vi "LsstLineDecode.vi"(11 "new lines":string) -> (0 "Chart":dbl(graph), 1 "payload":string, 2 "cmd":string, 3 "text":string, 4 "Graph":dbl[](graph))   [LabVIEW 2022 SP3]
uses:
  <vilib>/Utility/error.llb/Trim Whitespace One-Sided.vi
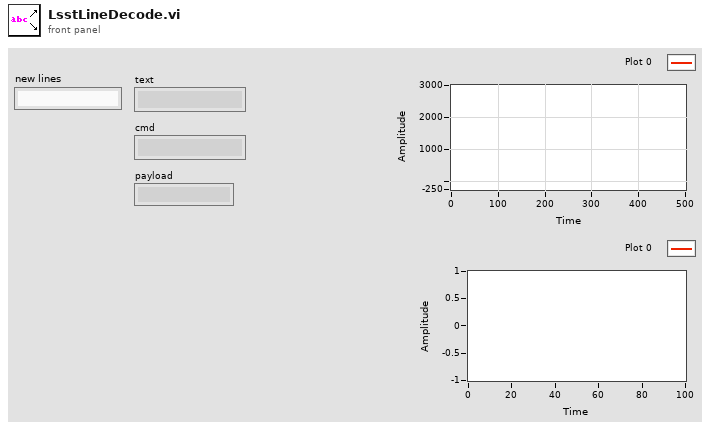
[diagram p1: front panel]
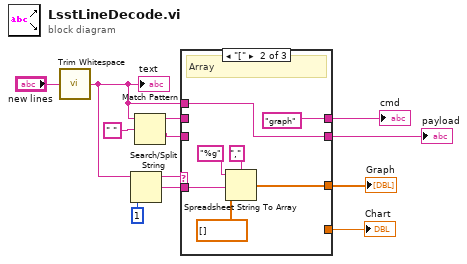
[diagram p0: block diagram]
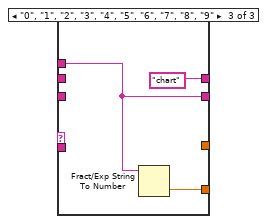
[diagram p3: hidden frame]
diagram:
  n1 = call <vilib>:"Trim Whitespace.vi"("string"="new lines") -> ("trimmed string"=w3:string)  [unwired: 1 in]
  "text" <- w3
  n2 = Search/Split String(string=w3, offset (0)=1) -> (substring before match=w5:string, match + rest of string=w4:string)  [unwired: 1 in, 1 out]
  n3 = Match Pattern(string=w3, regular expression=" ") -> (before substring=w9:string, after substring=w7:string)  [unwired: 1 in, 2 out]
  n4 = case shown="\"[\"" w5 {
    tunnel: w4 -> [_ w19 _]
    tunnel: [_ w17 _] -> w12
    tunnel: [w14 "graph" ("regular expression") "chart" ("regular expression")] -> w1
    tunnel: w9 -> [w14 _ _]
    tunnel: [w13 w15 w22] -> w8
    tunnel: w7 -> [w13 _ _]
    tunnel: w3 -> [_ w15 w22]
    tunnel: [_ _ w24] -> w2
    frame Default {
      # "not data"
    }
    frame "[" {
      # "Array"
      n5 = Spreadsheet String To Array(delimiter (Tab)=",", format string="%g", spreadsheet string=w19, array type (2D Dbl)=dbl[] []) -> (array=w17:dbl[])
    }
    frame "0", "1", "2", "3", "4", "5", "6", "7", "8", "9" {
      n6 = Fract/Exp String To Number(string=w22) -> (number=w24:dbl)  [unwired: 3 in, 1 out]
    }
  }
  "Graph" <- w12
  "Chart" <- w2
  "payload" <- w8
  "cmd" <- w1
